vi "PmuDelay.vi"() -> ()   [LabVIEW 2018, in "Visualization.lvlib" / "VisualizeAnalysis.lvclass"]
uses:
  VisualizeAnalysis.lvclass
  VisualizeBase/VisualizeBase_class/SubVIs/VisualizationOptions.ctl
  <vilib>/Utility/miscctls.llb/LVRectTypeDef.ctl
  VisualizeBase/VisualizeBase_class/Requests/VisUserEventType.ctl
  <vilib>/event_ctls.llb/usereventprio.ctl
  <extravilib>/ChannelInstances/Tag-bool/Write With Abort.vi
  <extravilib>/ChannelInstances/Tag-bool/Read With Abort.vi
  <extravilib>/ChannelInstances/Tag-bool/Instantiate.vi
  <extravilib>/ChannelInstances/Tag-bool/EndpointRead.vi
  <vilib>/Utility/error.llb/Error Cluster From Error Code.vi
  <extravilib>/ChannelInstances/Tag-bool/Endpoint.vi
  <vilib>/ErrorRing/Error Ring.xnode
  VisualizeBase/VisualizeBase_class/VisualizeBase.lvclass
  Analysis/AnalysisModule/AnalysisModule.lvlib
  <userlib>/NIST/NISTErrorLib/NISTErrorLib.lvlib
  StatusAndLog/VisualizeStatus.lvclass
  <extravilib>/ChannelInstances/Tag-bool.lvlib
panel:
  in  "Log Data":bool=TRUE
  in  "btnReset":bool
  out "ROCOF":cluster{"Freq":dbl, "Freq":dbl}[](graph)
  out "Freq":cluster{"Freq":dbl, "Freq":dbl}[](graph)
  in  "PluginName":string="Sensor.RoomAlert1"
  in  "btnClearTest":bool
  in  "btnPause":bool
  in  "btnOpen":bool
  in  "INIFilePath":path
  out "VisualizationProperties":T1={"PauseAtStartup"=TRUE, "LogData"=FALSE, "LaunchInSubPanel"=TRUE, "FPMonitor"=0, "FPWindowBounds"={"Left"=0, "Top"=0, "Right"=0, "Bottom"=0}, "MonitorBounds"={"Left"=0, "Top"=0, "Right"=0, "Bottom"=0}}
  in  "ModuleID":i32
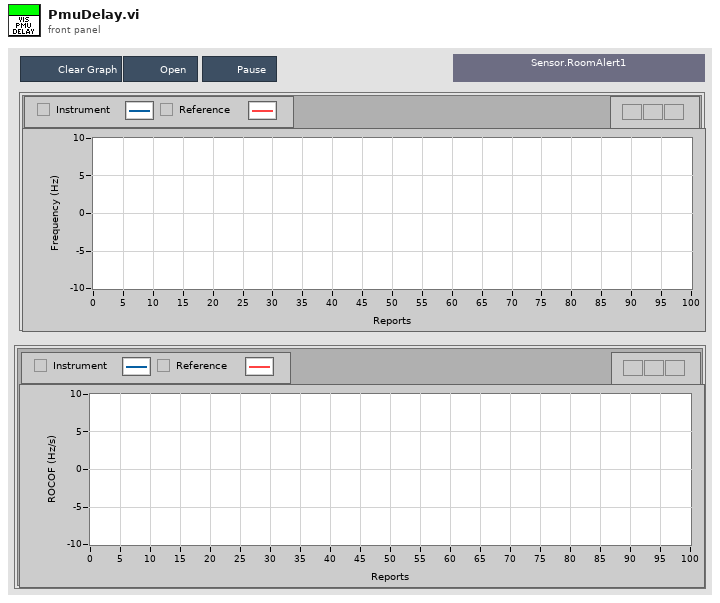
[diagram p1: front panel]
types:
  T1 = typedef "Visualization.lvlib/VisualizeBase.lvclass/VisualizationOptions.ctl" = cluster{"PauseAtStartup":bool, "LogData":bool, "LaunchInSubPanel":bool, "FPMonitor":u16, "FPWindowBounds":T2, "MonitorBounds":cluster{"Left":i16, "Top":i16, "Right":i16, "Bottom":i16}}
  T2 = typedef "LVRectTypeDef.ctl" = cluster{"Left":i16, "Top":i16, "Right":i16, "Bottom":i16}
  T3 = typedef "Visualization.lvlib/VisualizeBase.lvclass/VisRequestEvents.ctl" = cluster{"StopRequest":refnum<user-event>, "ResetRequest":refnum<user-event>, "FP Pop In or Out":refnum<user-event>}
  T4 = typedef "AnalysisModule.lvlib/clBroadcastEvents.ctl" = cluster{"DidInit":refnum<user-event>, "StatusUpdate":refnum<user-event>, "ErrorReport":refnum<user-event>, "DidStop":refnum<user-event>, "PathToINI":refnum<user-event>, "Config":refnum<user-event>, "ResultReport":refnum<user-event>, "FunctionClass":refnum<user-event>, "State":refnum<user-event>, "FunctionParams":refnum<user-event>, "Duration":refnum<user-event>}
  T5 = typedef "usereventprio.ctl" = enum32{"high priority", "normal priority"}
  T6 = typedef "Visualization.lvlib/VisualizeBase.lvclass/VisUserEventType.ctl" = cluster{"BusIndex":i8, "Data":variant}
  T7 = typedef "Tag-bool.lvlib/))Channel.ctl" = refnum<queue>
  T8 = typedef "sizeaction.ctl" = enum32{"Minimized", "Maximized", "Resized"}
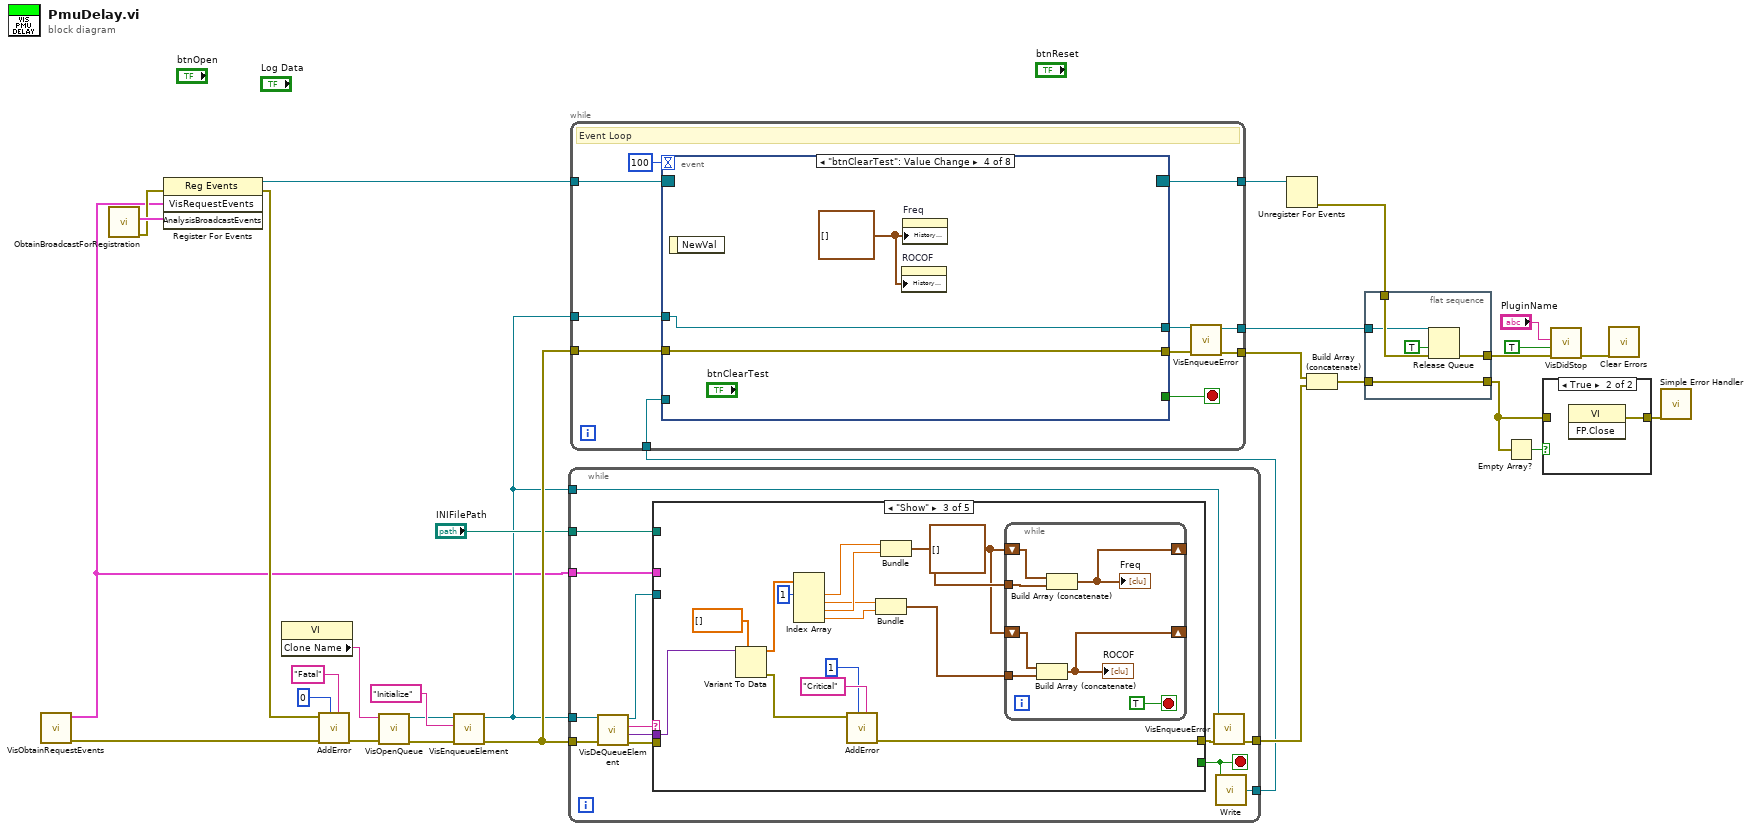
[diagram p0: block diagram]
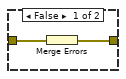
[diagram p2: hidden frame]
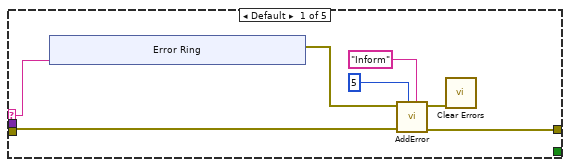
[diagram p3: hidden frame]
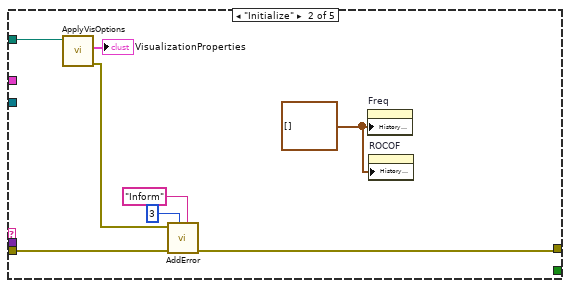
[diagram p4: hidden frame]
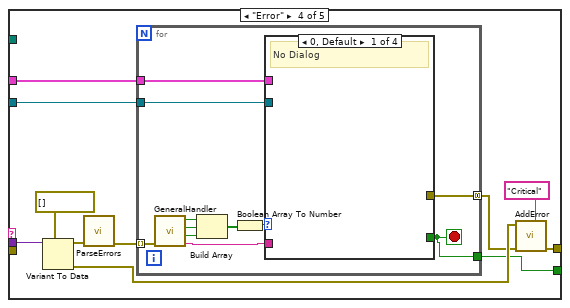
[diagram p5: hidden frame]
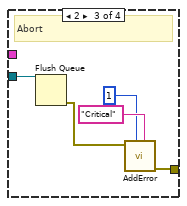
[diagram p7: hidden frame]
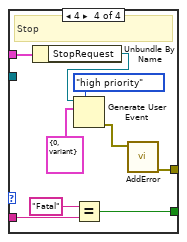
[diagram p8: hidden frame]
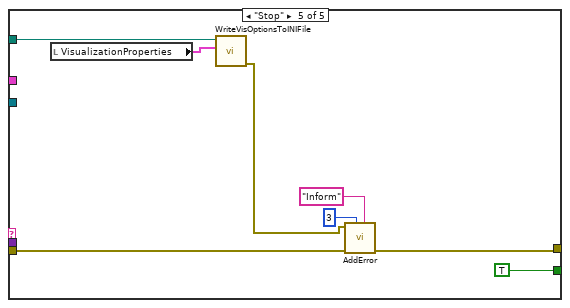
[diagram p9: hidden frame]
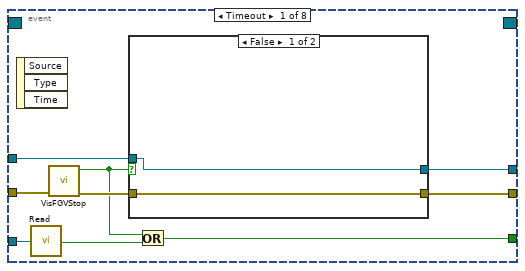
[diagram p10: hidden frame]
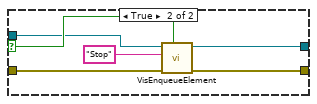
[diagram p11: hidden frame]
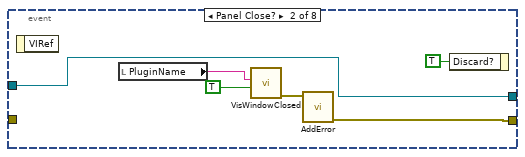
[diagram p12: hidden frame]
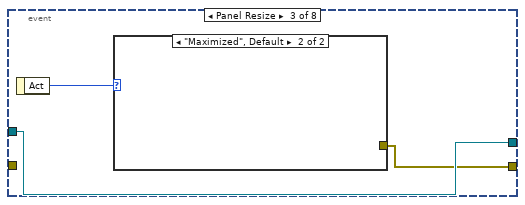
[diagram p13: hidden frame]
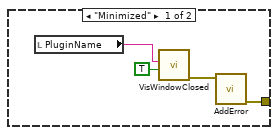
[diagram p14: hidden frame]
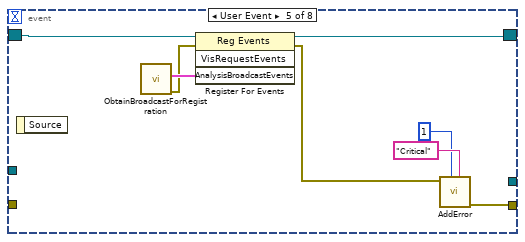
[diagram p15: hidden frame]
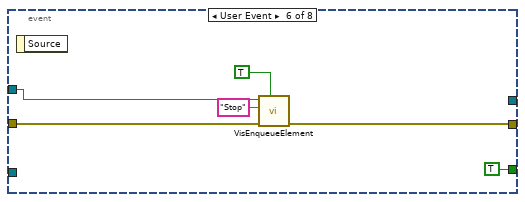
[diagram p16: hidden frame]
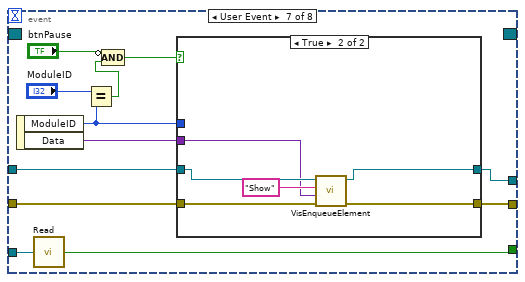
[diagram p17: hidden frame]
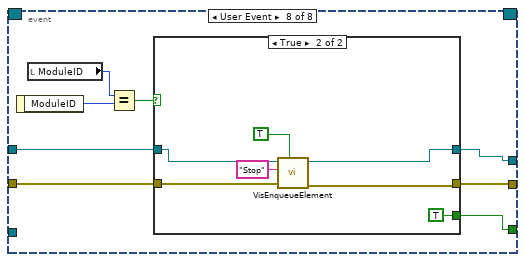
[diagram p19: hidden frame]
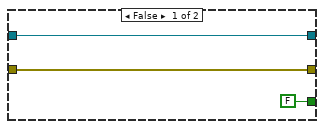
[diagram p20: hidden frame]
diagram:
  n1 = call "VisObtainRequestEvents.vi"() -> ("Error"=w29:errorcluster[], "VisRequestEvents"=w8:T3)  [unwired: 10 in]
  n2 = call "ObtainBroadcastForRegistration.vi"() -> ("error out"=w28:errorcluster, "AnalysisBroadcastEvents"=w30:T4)  [unwired: 10 in]
  n3 = register-events(error in=w28, w8, w30) -> (reference out=w20:refnum<event-registration>, error out=w27:errorcluster)  [unwired: 1 in]
  n4 = property class="VI"() -> ("Clone Name"=w22:string)  [unwired: 2 in, 2 out]
  n5 = call <userlib>:"AddError.vi"("Severity"="Fatal", "Priority"=u8 0, "ErrorArray In"=w29, "error in (no error)"=w27) -> ("ErrorArray Out"=w24:errorcluster[])  [unwired: 6 in, 1 out]
  n6 = call "VisOpenQueue.vi"("Error Array In"=w24, "QueueName"=w22) -> ("Error Array Out"=w23:errorcluster[], "queue out"=w19:refnum<queue>)  [unwired: 8 in]
  n7 = call "VisEnqueueElement.vi"("Error Array In"=w23, "Message"="Initialize", "queue in"=w19) -> ("Error Array Out"=w17:errorcluster[], "queue out"=w9:refnum<queue>)  [unwired: 7 in]
  n8 = while {
    tunnel: w17 -> [w43]
    tunnel: w9 -> [w42]
    tunnel: "INIFilePath" -> [w38]
    tunnel: [w34] -> w12
    tunnel: [w36] -> w10
    tunnel: w9 -> [w33]
    tunnel: w8 -> [w32]
    stop <- w37 stop-if-true
    n9 = call "VisDeQueueElement.vi"("Error Array In"=w43, "Queue In"=w42) -> ("Error Array Out"=w41:errorcluster[], "Data"=w40:variant, "Message"=w39:string, "Queue Out"=w31:refnum<queue>)  [unwired: 6 in]
    n10 = case shown="\"Show\"" w39 {
      selector: w39 -> [w44 _ _ _ _]
      tunnel: w41 -> [w46 w63 _ _ w129]
      tunnel: w40 -> [_ _ w80 w98 _]
      tunnel: w38 -> [_ w65 _ _ w131]
      tunnel: [w45 w59 w78 w93 w125] -> w35
      tunnel: [_ _ _ w90 TRUE] -> w37
      tunnel: w32 -> [_ _ _ w94 _]
      tunnel: w31 -> [_ _ _ w88 _]
      frame Default {
        n11 = xnode "Error Ring"("parameter 0"=w44) -> ("error out"=w50:errorcluster)
        n12 = call <userlib>:"AddError.vi"("Severity"="Inform" ("String"), "Priority"=u8 5, "ErrorArray In"=w46, "error in (no error)"=w50) -> ("ErrorArray Out"=w45:errorcluster[], "error out"=w49:errorcluster)  [unwired: 6 in]
        n13 = call <vilib>:"Clear Errors.vi"("error in (no error)"=w49) -> ()  [unwired: 5 in, 2 out]
      }
      frame "Initialize" {
        w58 = cluster{"Freq":dbl, "Freq":dbl}[] [] ("History Data")
        n14 = call "ApplyVisOptions.vi"("INIFilePath"=w65) -> ("error out"=w62:errorcluster, "VisualizationProperties"=→"VisualizationProperties":T1)  [unwired: 9 in]
        n15 = call <userlib>:"AddError.vi"("Severity"="Inform", "Priority"=u8 3, "ErrorArray In"=w63, "error in (no error)"=w62) -> ("ErrorArray Out"=w59:errorcluster[])  [unwired: 6 in, 1 out]
        n16 = property on="Freq" class="WFChart (strict)"("History Data"=w58) -> ()  [unwired: 2 in, 2 out]
        n17 = property on="ROCOF" class="WFChart (strict)"("History Data"=w58) -> ()  [unwired: 2 in, 2 out]
      }
      frame "Show" {
        w66 = cluster{"Freq":dbl, "Freq":dbl}[] []
        n18 = Variant To Data(type=dbl[] [], Variant=w80) -> (data=w74:dbl[], error out=w77:errorcluster)  [unwired: 1 in]
        n19 = Index Array(array=w74, index #1=1 ("index")) -> (element #1=w72:dbl, element #2=w70:dbl, element #3=w71:dbl, element #4=w69:dbl)  [unwired: 3 in]
        n20 = call <userlib>:"AddError.vi"("Severity"="Critical", "Priority"=u8 1, "error in (no error)"=w77) -> ("ErrorArray Out"=w78:errorcluster[])  [unwired: 7 in, 1 out]
        n21 = Bundle("Freq"=w70, "Freq"=w69) -> (w67:cluster{"Freq":dbl, "Freq":dbl})  [unwired: 1 in]
        n22 = Bundle("Freq"=w72, "Freq"=w71) -> (w68:cluster{"Freq":dbl, "Freq":dbl})  [unwired: 1 in]
        n23 = while {
          tunnel: w68 -> [w87]
          shift-right: [w85] -> _
          shift-left: w66 -> [w86]
          tunnel: w67 -> [w84]
          shift-right: [w83] -> _
          shift-left: w66 -> [w82]
          stop <- TRUE stop-if-true
          n24 = Build Array (concatenate)(w82, w84) -> (w83:cluster{"Freq":dbl, "Freq":dbl}[])
          "ROCOF" <- w83
          n25 = Build Array (concatenate)(w86, w87) -> (w85:cluster{"Freq":dbl, "Freq":dbl}[])
          "Freq" <- w85
        }
      }
      frame "Error" {
        n26 = Variant To Data(type=errorcluster[] [], Variant=w98) -> (data=w96:errorcluster[], error out=w92:errorcluster)  [unwired: 1 in]
        n27 = call <userlib>:"ParseErrors.vi"("ErrorArray"=w96) -> ("ErrorArray"=w95:errorcluster[])  [unwired: 8 in, 2 out]
        n28 = for {
          tunnel: w95 -> [w109] mode=indexing
          tunnel: w94 -> [w104]
          tunnel: [w101] -> w90
          tunnel: [w100] -> w89 mode=concatenating
          tunnel: w88 -> [w99]
          stop <- w101 stop-if-true
          n29 = call <userlib>:"GeneralHandler.vi"("error in (no error)"=w109) -> ("Severity"=w102:string, "Stop"=w108:bool, "Abort"=w107:bool, "Continue"=w106:bool)  [unwired: 6 in, 1 out]
          n30 = Build Array(w106, w107, w108) -> (w105:bool[])
          n31 = Boolean Array To Number(Boolean array=w105) -> (number=w103:u32)
          n32 = case shown="0, Default" w103 {
            tunnel: w104 -> [_ _ _ w123]
            tunnel: w102 -> [_ _ _ w119]
            tunnel: [_ _ _ w117] -> w101
            tunnel: [_ _ w113 w115] -> w100
            tunnel: w99 -> [_ _ w114 _]
            frame 0, Default {
              # "No Dialog"
            }
            frame 1 {
              # "Continue"
            }
            frame 2 {
              # "Abort"
              n33 = Flush Queue(queue=w114) -> (error out=w112:errorcluster)  [unwired: 1 in, 2 out]
              n34 = call <userlib>:"AddError.vi"("Severity"="Critical", "Priority"=u8 1, "error in (no error)"=w112) -> ("ErrorArray Out"=w113:errorcluster[])  [unwired: 7 in, 1 out]
            }
            frame 4 {
              # "Stop"
              n35 = Unbundle By Name(w123) -> ("StopRequest"=w121:refnum<user-event>)
              n36 = Generate User Event(priority (normal)=usereventprio."high priority", user event=w121, event data cluster=T6 {"BusIndex"=0, "Data"=variant} ("event data")) -> (error out=w116:errorcluster)  [unwired: 1 in, 1 out]
              n37 = Equal?(x="Fatal", y=w119) -> (x = y?=w117:bool)
              n38 = call <userlib>:"AddError.vi"("error in (no error)"=w116) -> ("ErrorArray Out"=w115:errorcluster[])  [unwired: 9 in, 1 out]
            }
          }
        }
        n39 = call <userlib>:"AddError.vi"("Severity"="Critical", "ErrorArray In"=w89, "error in (no error)"=w92) -> ("ErrorArray Out"=w93:errorcluster[])  [unwired: 7 in, 1 out]
      }
      frame "Stop" {
        n40 = local read "VisualizationProperties"() -> (w130:T1)
        n41 = call "WriteVisOptionsToINIFile.vi"("Visualization Options"=w130, "INIFilePath"=w131) -> ("error out"=w126:errorcluster)  [unwired: 8 in, 1 out]
        n42 = call <userlib>:"AddError.vi"("Severity"="Inform", "Priority"=u8 3, "ErrorArray In"=w129, "error in (no error)"=w126) -> ("ErrorArray Out"=w125:errorcluster[])  [unwired: 6 in, 1 out]
      }
    }
    n43 = call "VisEnqueueError.vi"("Error Array In"=w35, "Queue in"=w33) -> ("Error Array Out"=w34:errorcluster[])  [unwired: 8 in, 1 out]
    n44 = call <extravilib>:"Write.vi"("element"=w37) -> ("channel"=w36:T7)  [unwired: 1 out]
  }
  n45 = while {
    tunnel: w20 -> [w141]
    tunnel: w17 -> [w140]
    tunnel: w9 -> [w139]
    tunnel: [w135] -> w13
    tunnel: [w134] -> w15
    tunnel: [w133] -> w18
    tunnel: w10 -> [w132]
    stop <- w136 stop-if-true
    # "Event Loop"
    n46 = event shown="[3] \"btnClearTest\": Value Change" {
      selector: w141 -> [_ _ _ _ w183 _ _ _]
      dyn-events: [_ _ _ _ w180 _ _ _] -> w133
      timeout: 100 -> [_ _ _ _ _ _ _ _]
      tunnel: w140 -> [w151 _ _ w174 _ w189 w191 w213]
      tunnel: w139 -> [w149 w160 w168 w175 _ w185 w193 w214]
      tunnel: [w148 w160 w168 w175 _ _ w192 w212] -> w138
      tunnel: [w147 w163 w166 w174 w179 w186 w190 w211] -> w137
      tunnel: [w145 _ _ _ _ TRUE w200 w210] -> w136
      tunnel: w132 -> [w144 _ _ _ _ _ w201 _]
      event Timeout {
        n47 = event-data() -> ()  [unwired: 1 in, 3 out]
        n48 = call <extravilib>:"Read.vi"("channel"=w144) -> ("element"=w143:bool)  [unwired: 1 in, 1 out]
        n49 = call "VisFGVStop.vi"("Error In"=w151) -> ("Error Out"=w150:errorcluster[], "Value"=w146:bool)  [unwired: 9 in]
        n50 = case shown="False" w146 {
          selector: w146 -> [_ w157]
          tunnel: w150 -> [w153 w159]
          tunnel: w149 -> [w152 w156]
          tunnel: [w152 w155] -> w148
          tunnel: [w153 w154] -> w147
          frame False {
          }
          frame True {
            n51 = call "VisEnqueueElement.vi"("Priority? (F)"=w157, "Error Array In"=w159, "Message"="Stop", "queue in"=w156) -> ("Error Array Out"=w154:errorcluster[], "queue out"=w155:refnum<queue>)  [unwired: 6 in]
          }
        }
        n52 = Or(x=w146, y=w143) -> (x .or. y?=w145:bool)
      }
      event Panel Close? {
        n53 = event-data() -> ()  [unwired: 1 in, 1 out]
        n54 = local read "PluginName"() -> (w165:string)
        n55 = call "VisWindowClosed.vi"("Window Closed?"=TRUE, "Module Name"=w165) -> ("error out"=w162:errorcluster)  [unwired: 9 in]
        n56 = call <userlib>:"AddError.vi"("error in (no error)"=w162) -> ("ErrorArray Out"=w163:errorcluster[])  [unwired: 9 in, 1 out]
        n57 = event-data("Discard?"=TRUE) -> ()  [unwired: 1 in, 1 out]
      }
      event Panel Resize {
        n58 = event-data() -> ("Act"=w167:T8)  [unwired: 1 in]
        n59 = case shown="\"Maximized\", Default" w167 {
          tunnel: [w169 _] -> w166
          frame "Minimized" {
            n60 = local read "PluginName"() -> (w172:string)
            n61 = call "VisWindowClosed.vi"("Window Closed?"=TRUE, "Module Name"=w172) -> ("error out"=w170:errorcluster)  [unwired: 9 in]
            n62 = call <userlib>:"AddError.vi"("error in (no error)"=w170) -> ("ErrorArray Out"=w169:errorcluster[])  [unwired: 9 in, 1 out]
          }
          frame "Maximized", Default {
          }
        }
      }
      event "btnClearTest": Value Change {
        w173 = cluster{"Freq":dbl, "Freq":dbl}[] [] ("History Data")
        n63 = event-data() -> ()  [unwired: 1 in, 1 out]
        n64 = property on="ROCOF" class="WFChart (strict)"("History Data"=w173) -> ()  [unwired: 2 in, 2 out]
        n65 = property on="Freq" class="WFChart (strict)"("History Data"=w173) -> ()  [unwired: 2 in, 2 out]
      }
      event User Event {
        n66 = event-data() -> ()  [unwired: 1 in, 1 out]
        n67 = call "ObtainBroadcastForRegistration.vi"() -> ("error out"=w181:errorcluster, "AnalysisBroadcastEvents"=w182:T4)  [unwired: 10 in]
        n68 = register-events(reference=w183, error in=w181, w182) -> (reference out=w180:refnum<event-registration>, error out=w178:errorcluster)  [unwired: 1 in]
        n69 = call <userlib>:"AddError.vi"("Severity"="Critical", "Priority"=u8 1, "error in (no error)"=w178) -> ("ErrorArray Out"=w179:errorcluster[])  [unwired: 7 in, 1 out]
      }
      event User Event {
        n70 = event-data() -> ()  [unwired: 1 in, 1 out]
        n71 = call "VisEnqueueElement.vi"("Priority? (F)"=TRUE, "Error Array In"=w189, "Message"="Stop", "queue in"=w185) -> ("Error Array Out"=w186:errorcluster[])  [unwired: 6 in, 1 out]
      }
      event User Event {
        n72 = event-data() -> ("ModuleID"=w198:i32, "Data"=w199:variant)  [unwired: 1 in]
        n73 = call <extravilib>:"Read.vi"("channel"=w201) -> ("element"=w200:bool)  [unwired: 1 in, 1 out]
        n74 = Equal?(x="ModuleID", y=w198) -> (x = y?=w195:bool)
        n75 = Compound Arithmetic op=AND(invert "btnPause", w195) -> (w194:bool)
        n76 = case shown="True" w194 {
          tunnel: w198 -> [_ _]
          tunnel: w199 -> [_ w204]
          tunnel: [w203 w206] -> w192
          tunnel: w193 -> [w203 w208]
          tunnel: w191 -> [w202 w209]
          tunnel: [w202 w207] -> w190
          frame False {
          }
          frame True {
            n77 = call "VisEnqueueElement.vi"("Error Array In"=w209, "Data"=w204, "Message"="Show", "queue in"=w208) -> ("Error Array Out"=w207:errorcluster[], "queue out"=w206:refnum<queue>)  [unwired: 6 in]
          }
        }
      }
      event User Event {
        n78 = event-data() -> ("ModuleID"=w217:i32)  [unwired: 1 in]
        n79 = local read "ModuleID"() -> (w216:i32)
        n80 = Equal?(x=w216, y=w217) -> (x = y?=w215:bool)
        n81 = case shown="True" w215 {
          tunnel: w214 -> [w220 w226]
          tunnel: w213 -> [w219 w227]
          tunnel: [w220 w224] -> w212
          tunnel: [w219 w225] -> w211
          tunnel: [FALSE TRUE] -> w210
          frame False {
          }
          frame True {
            n82 = call "VisEnqueueElement.vi"("Priority? (F)"=TRUE, "Error Array In"=w227, "Message"="Stop", "queue in"=w226) -> ("Error Array Out"=w225:errorcluster[], "queue out"=w224:refnum<queue>)  [unwired: 6 in]
          }
        }
      }
    }
    n83 = call "VisEnqueueError.vi"("Error Array In"=w137, "Queue in"=w138) -> ("Error Array Out"=w135:errorcluster[], "Queue out"=w134:refnum<queue>)  [unwired: 8 in]
  }
  n84 = Unregister For Events(event registration refnum=w18) -> (error out=w16:errorcluster)  [unwired: 1 in]
  n85 = Build Array (concatenate)(w13, w12) -> (w11:errorcluster[])
  n86 = flat-sequence {
    tunnel: w16 -> [w232]
    tunnel: w15 -> [w230]
    tunnel: [w229] -> w2
    tunnel: w11 -> [w229]
    tunnel: [w228] -> w7
    frame #0 {
      n87 = Release Queue(queue=w230, force destroy? (F)=TRUE, error in (no error)=w232) -> (error out=w228:errorcluster)  [unwired: 2 out]
    }
  }
  n88 = Empty Array?(array=w2) -> (empty?=w4:bool)
  n89 = case shown="True" w4 {
    tunnel: w2 -> [w234 _]
    tunnel: [w233 w235] -> w1
    frame False {
      n90 = Merge Errors(w234) -> (w233:errorcluster)
    }
    frame True {
      n91 = invoke class="VI" method="FP.Close"() -> (error out=w235:errorcluster)  [unwired: 3 in, 2 out]
    }
  }
  n92 = call "VisDidStop.vi"("error in (no error)"=w7, "DidStop?"=TRUE, "Module Name"="PluginName") -> ("error out"=w3:errorcluster)  [unwired: 8 in]
  n93 = call <vilib>:"Clear Errors.vi"("error in (no error)"=w3) -> ()  [unwired: 5 in, 2 out]
  n94 = call <vilib>:"Simple Error Handler.vi"("error in (no error)"=w1) -> ()  [unwired: 4 in, 5 out]
